vi "Lang Set Desc.vi"(8 "error in (no error)":errorcluster, 10 "UI Descriptions":T1, 11 "LF2R IDE in":refnum<class "Main Panel.lvclass">) -> (0 "error out":errorcluster, 3 "LF2R IDE out":refnum<class "Main Panel.lvclass">)   [LabVIEW 2018, in "Framework.lvlib" / "Framework.lvclass"]
uses:
  Framework/Framework/Framework.lvclass
  Main Panel.lvclass
  Const Lang Property.ctl
  Const UI Desc Frame Basic.ctl
  Const UI Desc Frame Skill.ctl
  Const UI Desc Frame bp.ctl
  Const UI Desc Frame w.ctl
  Const UI Desc Frame Title.ctl
  Const UI Desc Frame b.ctl
  Const UI Desc Frame i.ctl
  Const UI Desc Frame o.ctl
  Const UI Desc Frame c.ctl
  Const Lang Setting.ctl
  Const UI Desc Other.ctl
  Const UI Desc Menu.ctl
  Const Lang CfgWnd Tab.ctl
  Const Lang CfgWnd Main.ctl
  Const Lang CfgWnd Path.ctl
  Framework/Framework/Const Lang CfgWnd Image.ctl
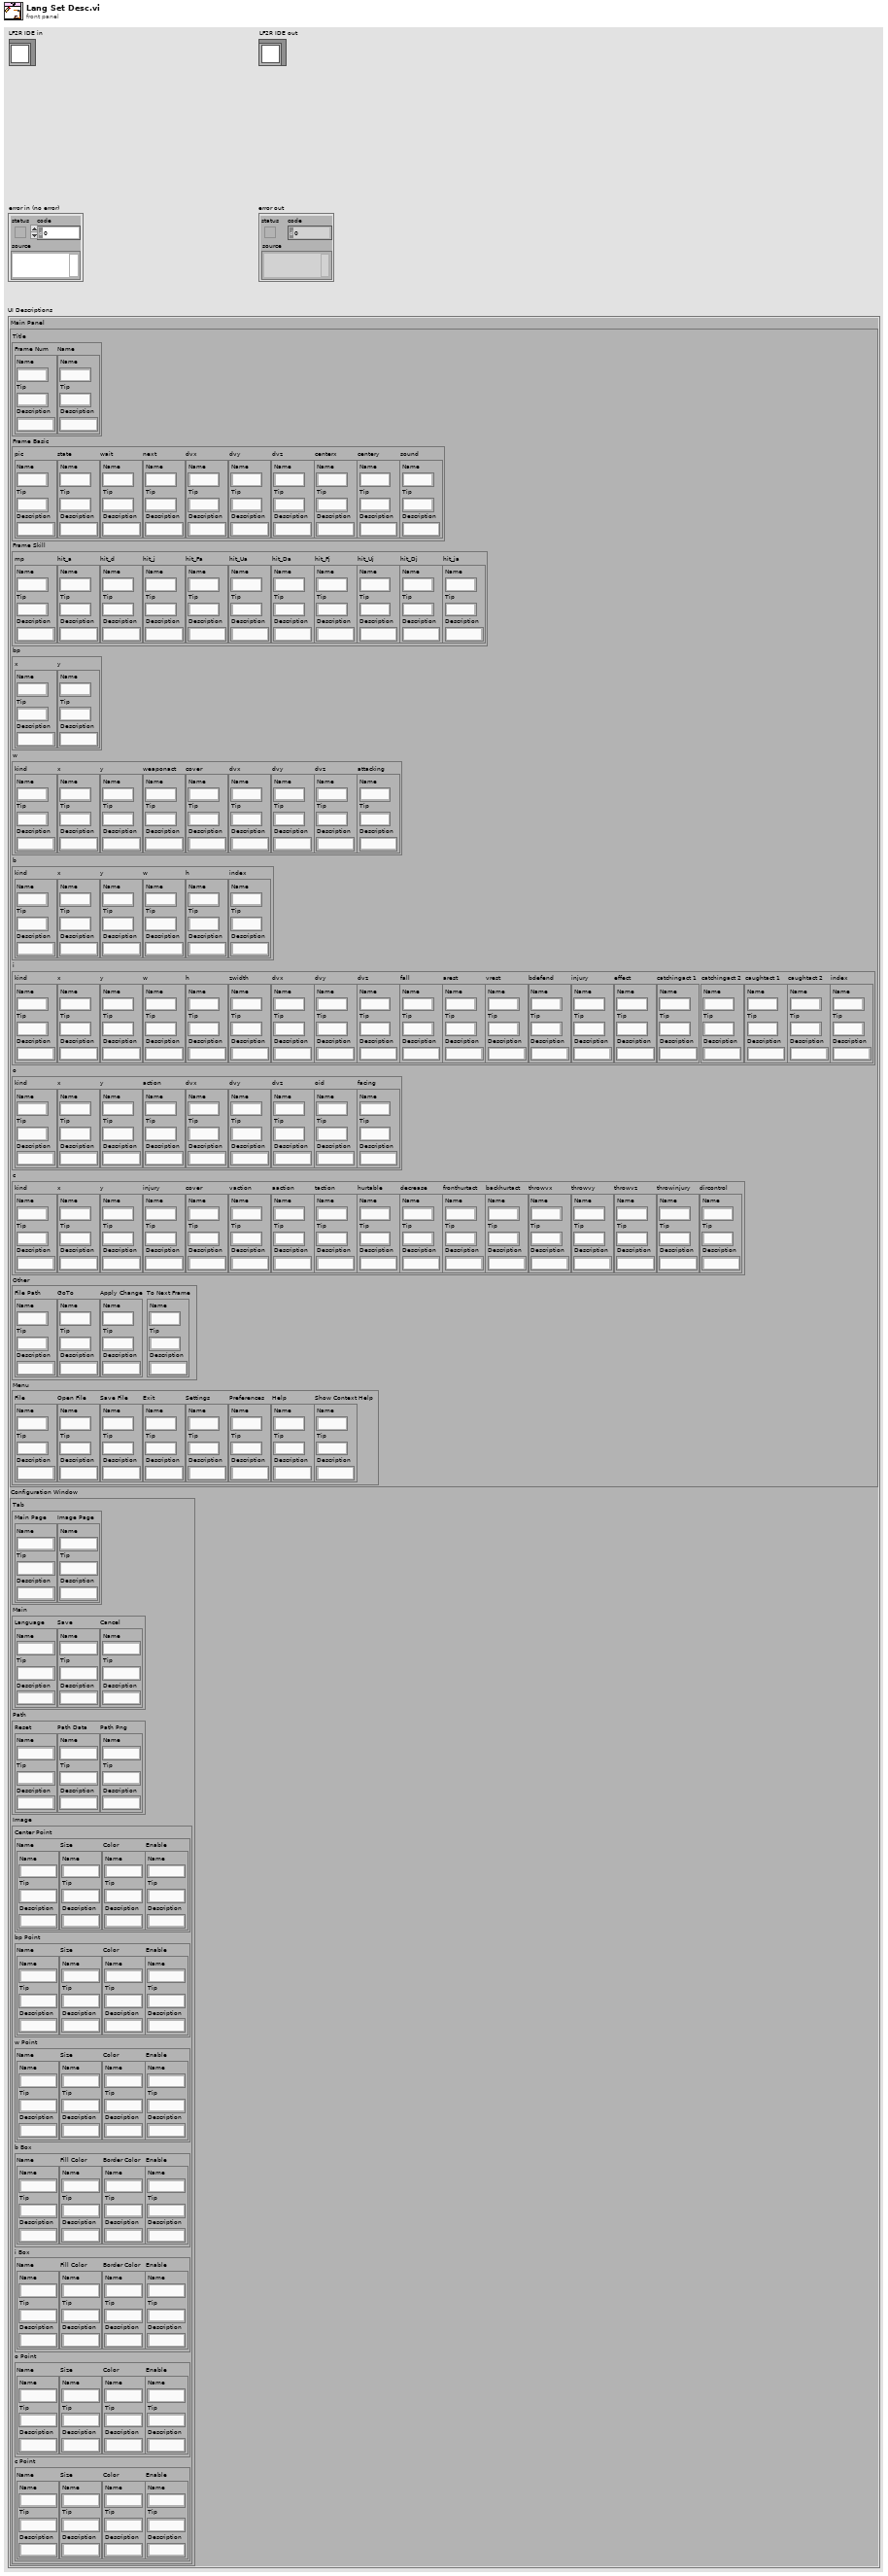
[diagram p1: front panel]
types:
  T1 = typedef "Framework.lvlib/Framework.lvclass/Const Lang Setting.ctl" = cluster{"Main Panel":cluster{"Title":T2, "Frame Basic":T4, "Frame Skill":T5, "bp":T6, "w":T7, "b":T8, "i":T9, "o":T10, "c":T11, "Other":T12, "Menu":T13}, "Configuration Window":cluster{"Tab":T14, "Main":T15, "Path":T16, "Image":T17}}
  T2 = typedef "Framework.lvlib/Framework.lvclass/Const UI Desc Frame Title.ctl" = cluster{"Frame Num":T3, "Name":T3}
  T3 = typedef "Framework.lvlib/Framework.lvclass/Const Lang Property.ctl" = cluster{"Name":string, "Tip":string, "Description":string}
  T4 = typedef "Framework.lvlib/Framework.lvclass/Const UI Desc Frame Basic.ctl" = cluster{"pic":T3, "state":T3, "wait":T3, "next":T3, "dvx":T3, "dvy":T3, "dvz":T3, "centerx":T3, "centery":T3, "sound":T3}
  T5 = typedef "Framework.lvlib/Framework.lvclass/Const UI Desc Frame Skill.ctl" = cluster{"mp":T3, "hit_a":T3, "hit_d":T3, "hit_j":T3, "hit_Fa":T3, "hit_Ua":T3, "hit_Da":T3, "hit_Fj":T3, "hit_Uj":T3, "hit_Dj":T3, "hit_ja":T3}
  T6 = typedef "Framework.lvlib/Framework.lvclass/Const UI Desc Frame bp.ctl" = cluster{"x":T3, "y":T3}
  T7 = typedef "Framework.lvlib/Framework.lvclass/Const UI Desc Frame w.ctl" = cluster{"kind":T3, "x":T3, "y":T3, "weaponact":T3, "cover":T3, "dvx":T3, "dvy":T3, "dvz":T3, "attacking":T3}
  T8 = typedef "Framework.lvlib/Framework.lvclass/Const UI Desc Frame b.ctl" = cluster{"kind":T3, "x":T3, "y":T3, "w":T3, "h":T3, "index":T3}
  T9 = typedef "Framework.lvlib/Framework.lvclass/Const UI Desc Frame i.ctl" = cluster{"kind":T3, "x":T3, "y":T3, "w":T3, "h":T3, "zwidth":T3, "dvx":T3, "dvy":T3, "dvz":T3, "fall":T3, "arest":T3, "vrest":T3, "bdefend":T3, "injury":T3, "effect":T3, "catchingact 1":T3, "catchingact 2":T3, "caughtact 1":T3, "caughtact 2":T3, "index":T3}
  T10 = typedef "Framework.lvlib/Framework.lvclass/Const UI Desc Frame o.ctl" = cluster{"kind":T3, "x":T3, "y":T3, "action":T3, "dvx":T3, "dvy":T3, "dvz":T3, "oid":T3, "facing":T3}
  T11 = typedef "Framework.lvlib/Framework.lvclass/Const UI Desc Frame c.ctl" = cluster{"kind":T3, "x":T3, "y":T3, "injury":T3, "cover":T3, "vaction":T3, "aaction":T3, "taction":T3, "hurtable":T3, "decrease":T3, "fronthurtact":T3, "backhurtact":T3, "throwvx":T3, "throwvy":T3, "throwvz":T3, "throwinjury":T3, "dircontrol":T3}
  T12 = typedef "Framework.lvlib/Framework.lvclass/Const UI Desc Other.ctl" = cluster{"File Path":T3, "GoTo":T3, "Apply Change":T3, "To Next Frame":T3}
  T13 = typedef "Framework.lvlib/Framework.lvclass/Const UI Desc Menu.ctl" = cluster{"File":T3, "Open File":T3, "Save File":T3, "Exit":T3, "Settings":T3, "Preferences":T3, "Help":T3, "Show Context Help":T3}
  T14 = typedef "Framework.lvlib/Framework.lvclass/Const Lang CfgWnd Tab.ctl" = cluster{"Main Page":T3, "Image Page":T3}
  T15 = typedef "Framework.lvlib/Framework.lvclass/Const Lang CfgWnd Main.ctl" = cluster{"Language":T3, "Save":T3, "Cancel":T3}
  T16 = typedef "Framework.lvlib/Framework.lvclass/Const Lang CfgWnd Path.ctl" = cluster{"Reset":T3, "Path Data":T3, "Path Png":T3}
  T17 = typedef "Framework.lvlib/Framework.lvclass/Const Lang CfgWnd Image.ctl" = cluster{"Center Point":cluster{"Name":T3, "Size":T3, "Color":T3, "Enable":T3}, "bp Point":cluster{"Name":T3, "Size":T3, "Color":T3, "Enable":T3}, "w Point":cluster{"Name":T3, "Size":T3, "Color":T3, "Enable":T3}, "b Box":cluster{"Name":T3, "Fill Color":T3, "Border Color":T3, "Enable":T3}, "i Box":cluster{"Name":T3, "Fill Color":T3, "Border Color":T3, "Enable":T3}, "o Point":cluster{"Name":T3, "Size":T3, "Color":T3, "Enable":T3}, "c Point":cluster{"Name":T3, "Size":T3, "Color":T3, "Enable":T3}}
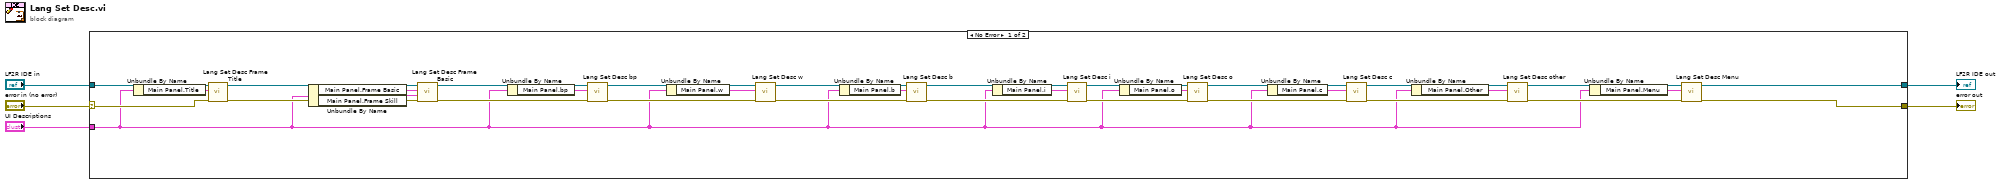
[diagram p0: block diagram]
diagram:
  n1 = case shown="No Error" "error in (no error)" {
    selector: "error in (no error)" -> [w37 w41]
    tunnel: [w8 w41] -> w4
    tunnel: [w9 w40] -> w2
    tunnel: "LF2R IDE in" -> [w39 w40]
    tunnel: "UI Descriptions" -> [w7 _]
    frame No Error {
      n2 = Unbundle By Name(w7) -> ("Main Panel.Title"=w38:T2)
      n3 = call "Lang Set Desc Frame Title.vi"("error in (no error)"=w37, "Title"=w38, "LF2R IDE in"=w39) -> ("error out"=w35:errorcluster, "LF2R IDE out"=w36:refnum<class "Main Panel.lvclass">)  [unwired: 7 in]
      n4 = Unbundle By Name(w7) -> ("Main Panel.Frame Basic"=w34:T4, "Main Panel.Frame Skill"=w33:T5)
      n5 = call "Lang Set Desc Frame Basic.vi"("error in (no error)"=w35, "Frame Skill"=w33, "Frame Basic"=w34, "LF2R IDE in"=w36) -> ("error out"=w31:errorcluster, "LF2R IDE out"=w32:refnum<class "Main Panel.lvclass">)  [unwired: 6 in]
      n6 = Unbundle By Name(w7) -> ("Main Panel.bp"=w30:T6)
      n7 = call "Lang Set Desc bp.vi"("error in (no error)"=w31, "bp"=w30, "LF2R IDE in"=w32) -> ("error out"=w28:errorcluster, "LF2R IDE out"=w29:refnum<class "Main Panel.lvclass">)  [unwired: 7 in]
      n8 = Unbundle By Name(w7) -> ("Main Panel.w"=w27:T7)
      n9 = call "Lang Set Desc w.vi"("error in (no error)"=w28, "w"=w27, "LF2R IDE in"=w29) -> ("error out"=w25:errorcluster, "LF2R IDE out"=w26:refnum<class "Main Panel.lvclass">)  [unwired: 7 in]
      n10 = Unbundle By Name(w7) -> ("Main Panel.b"=w24:T8)
      n11 = call "Lang Set Desc b.vi"("error in (no error)"=w25, "b"=w24, "LF2R IDE in"=w26) -> ("error out"=w22:errorcluster, "LF2R IDE out"=w23:refnum<class "Main Panel.lvclass">)  [unwired: 7 in]
      n12 = Unbundle By Name(w7) -> ("Main Panel.i"=w21:T9)
      n13 = call "Lang Set Desc i.vi"("error in (no error)"=w22, "i"=w21, "LF2R IDE in"=w23) -> ("error out"=w19:errorcluster, "LF2R IDE out"=w20:refnum<class "Main Panel.lvclass">)  [unwired: 7 in]
      n14 = Unbundle By Name(w7) -> ("Main Panel.o"=w16:T10)
      n15 = call "Lang Set Desc o.vi"("error in (no error)"=w19, "o"=w16, "LF2R IDE in"=w20) -> ("error out"=w17:errorcluster, "LF2R IDE out"=w18:refnum<class "Main Panel.lvclass">)  [unwired: 7 in]
      n16 = Unbundle By Name(w7) -> ("Main Panel.c"=w15:T11)
      n17 = call "Lang Set Desc c.vi"("error in (no error)"=w17, "c"=w15, "LF2R IDE in"=w18) -> ("error out"=w13:errorcluster, "LF2R IDE out"=w14:refnum<class "Main Panel.lvclass">)  [unwired: 7 in]
      n18 = Unbundle By Name(w7) -> ("Main Panel.Other"=w12:T12)
      n19 = call "Lang Set Desc other.vi"("error in (no error)"=w13, "Other"=w12, "LF2R IDE in"=w14) -> ("error out"=w10:errorcluster, "LF2R IDE out"=w11:refnum<class "Main Panel.lvclass">)  [unwired: 7 in]
      n20 = Unbundle By Name(w7) -> ("Main Panel.Menu"=w6:T13)
      n21 = call "Lang Set Desc Menu.vi"("error in (no error)"=w10, "Menu"=w6, "LF2R IDE in"=w11) -> ("error out"=w8:errorcluster, "LF2R IDE out"=w9:refnum<class "Main Panel.lvclass">)  [unwired: 7 in]
    }
    frame Error {
    }
  }
  "error out" <- w4
  "LF2R IDE out" <- w2
